vi "Do.vi"(8 "error in (no error)":errorcluster, 10 "Actor in":refnum<class "Actor.lvclass">, 11 "Conceret Edit Test Node List Msg in":refnum<class "Conceret Edit Test Node List Msg.lvclass">) -> (0 "error out":errorcluster, 2 "Actor out":refnum<class "Actor.lvclass">)   [LabVIEW 2013, in "Edit Test Node View.lvlib" / "Conceret Edit Test Node List Msg.lvclass"]
doc: "(<B>Filename</B>: Actor Framework.lvlib:Message.lvclass:Do.vi)\n\nDefines what a message does when it is received by an actor. Generally, a message instructs an actor to invoke one of its methods.\n\nBy default, this method does nothing. A child class must override it to define behavior. Create a child class by using the Actor Framework Message Maker dialog box."
uses:
  Conceret Edit Test Node List Msg.lvclass
  <vilib>/ActorFramework/Actor/Actor.lvclass
  Edit Test Node View/Edit Test Node View.lvclass
  Models/Edit Test Node Model Messages/Abstract Edit Test Node List Msg/Abstract Edit Test Node List Msg.lvclass
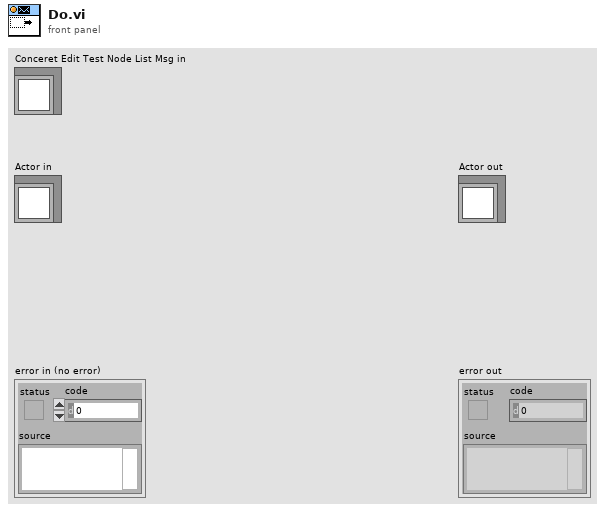
[diagram p1: front panel]
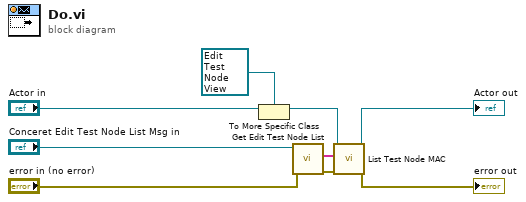
[diagram p0: block diagram]
diagram:
  n1 = To More Specific Class(target class=refnum<class "Edit Test Node View.lvclass"> refnum ("Edit Test Node View.lvlib:Edit Test Node View.lvclass"), reference="Actor in") -> (specific class reference=w6:refnum<class "Edit Test Node View.lvclass">)  [unwired: 1 in, 1 out]
  n2 = call "Get Edit Test Node List.vi"("error in (no error)"="error in (no error)", "Abstract Edit Test Node List Msg in"="Conceret Edit Test Node List Msg in") -> ("error out"=w5:errorcluster, "Edit Test Node List"=w1:string[])  [unwired: 7 in, 1 out]
  n3 = call "List Test Node MAC.vi"("error in (no error)"=w5, "Edit Test Node List"=w1, "Edit Test Node View in"=w6) -> ("error out"=→"error out":errorcluster, "Edit Test Node View out"=→"Actor out":refnum<class "Edit Test Node View.lvclass">)  [unwired: 7 in]
